vi "0x03ReadHoldingRegisters.vi"(6 "Length 2":u16, 8 "error in (no error)":errorcluster, 9 "Register":u16, 10 "Addressc":u8, 11 "RTU in":refnum<class "RTU.lvclass">) -> (0 "error out":errorcluster, 2 "Frame":string, 3 "RTU out":refnum<class "RTU.lvclass">)   [LabVIEW 2015, in "ModBUS.lvlib" / "RTU.lvclass"]
uses:
  RTU.lvclass
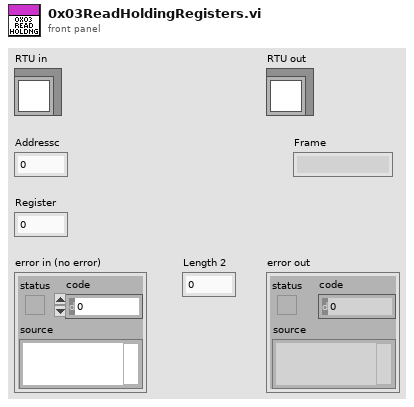
[diagram p1: front panel]
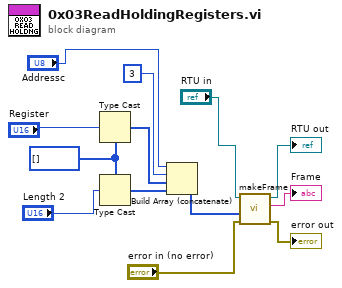
[diagram p0: block diagram]
diagram:
  w6 = u8[] []
  n1 = Type Cast(type=w6, x="Register") -> (*(type *) &x=w7:u8[])
  n2 = Type Cast(type=w6, x="Length 2") -> (*(type *) &x=w5:u8[])
  n3 = Build Array (concatenate)("Addressc", u8 3 ("element"), w7, w5) -> (w1:u8[])
  n4 = call-dynamic "makeFrame.vi"("error in (no error)"="error in (no error)", "Data"=w1, "RTU in"="RTU in") -> ("error out"=→"error out":errorcluster, "Frame"=→"Frame":string, "RTU out"=→"RTU out":refnum<class "RTU.lvclass">)  [unwired: 6 in]
